vi "Arquivo - Leitura.vi"() -> ()   [LabVIEW 2021]
panel:
  out "text":string
  out "path":path
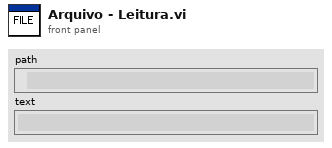
[diagram p1: front panel]
types:
  T1 = enum16{"open", "replace", "create", "open or create", "replace or create", "replace or create with confirmation"}
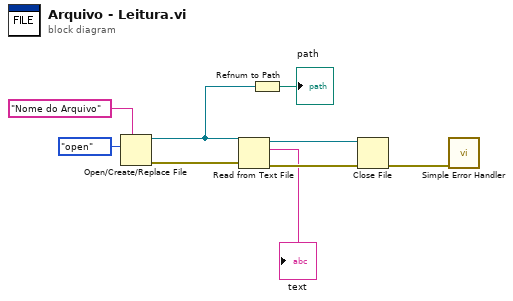
[diagram p0: block diagram]
diagram:
  n1 = Open/Create/Replace File(prompt="Nome do Arquivo", operation (0:open)=T1."open") -> (refnum out=w3:refnum<file>, error out=w8:errorcluster)  [unwired: 4 in, 1 out]
  n2 = Read from Text File(file (use dialog)=w3, error in=w8) -> (refnum out=w9:refnum<file>, text=→"text":string, error out=w7:errorcluster)  [unwired: 2 in, 1 out]
  n3 = Refnum to Path(1:w3) -> (0:→"path":path)
  n4 = Close File(refnum=w9, error in=w7) -> (error out=w6:errorcluster)  [unwired: 1 out]
  n5 = call <vilib>:"Simple Error Handler.vi"("error in (no error)"=w6) -> ()  [unwired: 4 in, 5 out]
